vi "Filter - Moving Point Average.vi"(9 "Analog Signal":dbl[](array[numeric])) -> (1 "Filtered Analog Signal":dbl[](array[numeric]))   [LabVIEW 2017, in "AI.lvclass"]
uses:
  AI.lvclass
  <vilib>/Analysis/baseanly.llb/Mean (DBL).vi
  <vilib>/Analysis/NI_AALBase.lvlib
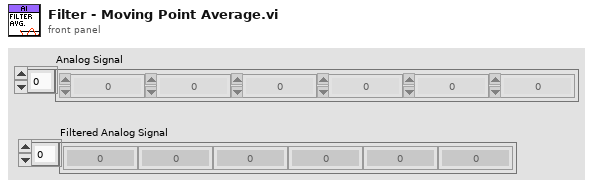
[diagram p1: front panel]
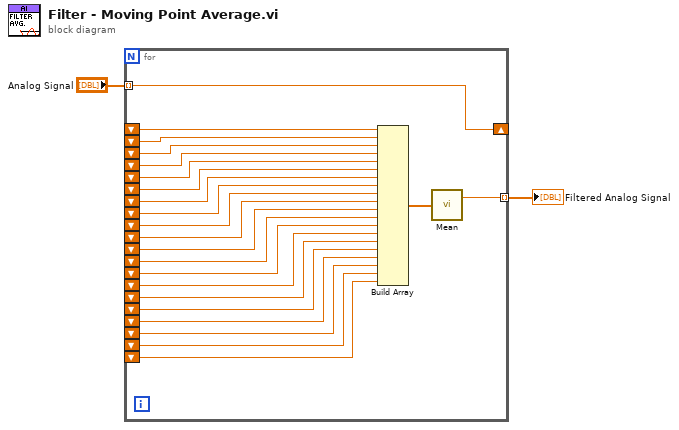
[diagram p0: block diagram]
diagram:
  n1 = for {
    shift-right: [w23] -> _
    shift-left: _ -> [w25]
    shift-left: _ -> [w24]
    shift-left: _ -> [w22]
    shift-left: _ -> [w21]
    shift-left: _ -> [w20]
    shift-left: _ -> [w19]
    shift-left: _ -> [w18]
    shift-left: _ -> [w17]
    shift-left: _ -> [w16]
    shift-left: _ -> [w15]
    tunnel: "Analog Signal" -> [w23] mode=indexing
    tunnel: [w13] -> w1 mode=indexing
    shift-left: _ -> [w12]
    shift-left: _ -> [w11]
    shift-left: _ -> [w10]
    shift-left: _ -> [w9]
    shift-left: _ -> [w8]
    shift-left: _ -> [w7]
    shift-left: _ -> [w6]
    shift-left: _ -> [w5]
    shift-left: _ -> [w4]
    shift-left: _ -> [w3]
    n2 = Build Array(w25, w24, w22, w21, w20, w19, w18, w17, w16, w15, w12, w11, w10, w9, w8, w7, w6, w5, w4, w3) -> (w14:dbl[])
    n3 = call-poly <vilib>:"Mean.vi"("X"=w14) -> ("mean"=w13:dbl)  [unwired: 1 out]
  }
  "Filtered Analog Signal" <- w1
